vi "default_configuration.vi"(8 "error in (no error)":errorcluster, 11 "project_file":string) -> (0 "error out":errorcluster, 3 "configuration":T1)   [LabVIEW 2015, in "lv-builder-default.lvlib"]
uses:
  lv-builder-default.lvlib
  public/_controls/configuration.ctl
  public/_controls/post_action_lvlib.ctl
  public/_controls/post_action_installer.ctl
  public/_controls/post_action_application.ctl
  public/_controls/post_action_zip.ctl
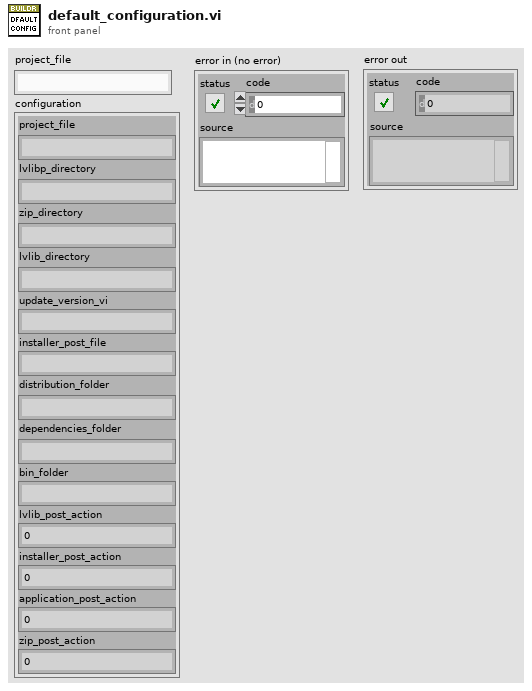
[diagram p1: front panel]
types:
  T1 = typedef "lv-builder-default.lvlib/configuration.ctl" = cluster{"project_file":string, "lvlibp_directory":string, "zip_directory":string, "lvlib_directory":string, "update_version_vi":string, "installer_post_file":string, "distribution_folder":string, "dependencies_folder":string, "bin_folder":string, "lvlib_post_action":u16, "installer_post_action":u16, "application_post_action":u16, "zip_post_action":u16}
  T2 = typedef "lv-builder-default.lvlib/post_action_zip.ctl" = enum16{"<zip_post_action>", "nothing", "move", "extract", "<null>"}
  T3 = typedef "lv-builder-default.lvlib/post_action_application.ctl" = enum16{"<application_post_action>", "nothing", "zip_application", "<null>"}
  T4 = typedef "lv-builder-default.lvlib/post_action_installer.ctl" = enum16{"<installer_post_action>", "nothing", "create_installer", "zip_installer", "create_installer_file", "<null>"}
  T5 = typedef "lv-builder-default.lvlib/post_action_lvlib.ctl" = enum16{"<lvlib_post_action>", "nothing", "move", "install", "<null>"}
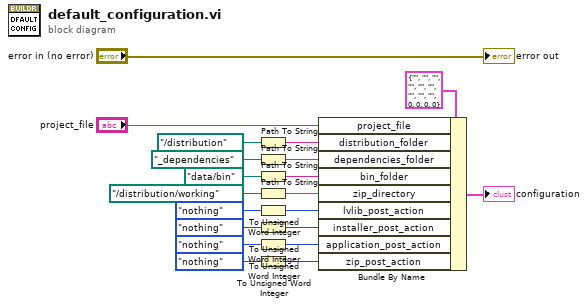
[diagram p0: block diagram]
diagram:
  n1 = Path To String(path=path "../distribution" ("appended path")) -> (string=w13:string)
  n2 = Path To String(path=path "_dependencies" ("appended path")) -> (string=w17:string)
  n3 = Path To String(path=path "data/bin" ("appended path")) -> (string=w15:string)
  n4 = Path To String(path=path "../distribution/working" ("appended path")) -> (string=w1:string)
  n5 = To Unsigned Word Integer(number=post_action_lvlib."nothing" ("lvlib_post_action")) -> (unsigned 16bit integer=w8:u16)
  n6 = To Unsigned Word Integer(number=post_action_installer."nothing" ("installer_post_action")) -> (unsigned 16bit integer=w7:u16)
  n7 = To Unsigned Word Integer(number=post_action_application."nothing" ("application_post_action")) -> (unsigned 16bit integer=w6:u16)
  n8 = To Unsigned Word Integer(number=post_action_zip."nothing" ("zip_post_action")) -> (unsigned 16bit integer=w5:u16)
  n9 = Bundle By Name(cluster=T1 {"project_file"="", "lvlibp_directory"="", "zip_directory"="", "lvlib_directory"="", "update_version_vi"="", "installer_post_file"="", "distribution_folder"="", "dependencies_folder"="", "bin_folder"="", "lvlib_post_action"=0, "installer_post_action"=0, "application_post_action"=0, "zip_post_action"=0} ("configuration"), "project_file"="project_file", "distribution_folder"=w13, "dependencies_folder"=w17, "bin_folder"=w15, "zip_directory"=w1, "lvlib_post_action"=w8, "installer_post_action"=w7, "application_post_action"=w6, "zip_post_action"=w5) -> (→"configuration":T1)
  "error out" <- "error in (no error)"
